vi "lxw version.vi"(8 "error in (no error)":errorcluster) -> (0 "error out":errorcluster, 3 "function return":string)   [LabVIEW 8.6]
doc: "const char* lxw_version(void);"
uses:
  pending_lvxlsxwriter/xlsxwriter.dll
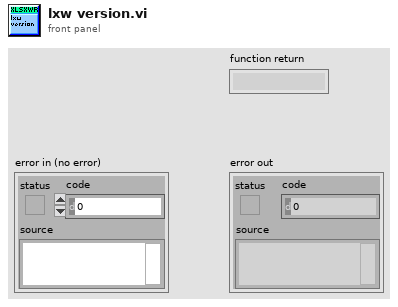
[diagram p1: front panel]
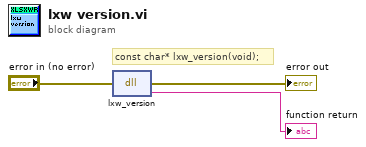
[diagram p0: block diagram]
diagram:
  # "const char* lxw_version(void);"
  n1 = dll-call lib="C:/Users/WDAGUtilityAccount/Desktop/pending_lvxlsxwriter/xlsxwriter.*" fn="lxw_version"(error in="error in (no error)") -> (error out=→"error out":errorcluster, →"function return":string)  [unwired: 2 in, 1 out]
